vi "MT Detect FSK.vi"(5 "input complex waveform":T3={"t0"=0.0, "dt"=1.0, "Y"=[]} {"Y" format="%.3f"; "dt" format="%^.2e"; "t0" format="%.4f"}, 7 "FSK system parameters":T2={"samples per symbol (16)"=16, "symbol map"=[], "symbol phase continuity"=enum."continuous"} {"symbol map" format="%.2f"}, 9 "synchronization parameters":T1 {"sync sequence" format="%.2f"}, 11 "error in (no error)":errorcluster, 12 "matched filter coefficients":dbl[](array[numeric]) format="%.2f", 13 "reset? (T)":bool=TRUE, 14 "flush buffers? (F)":bool) -> (6 "output bit stream":i8[](array[numeric]), 10 "sync found index (symbols)":dbl format="%.4f", 15 "error out":errorcluster)   [LabVIEW 2020, in "niDMT.lvlib"]
doc: "Demodulates a frequency-shift keying (FSK)-modulated complex baseband waveform and returns the demodulated information bit stream. This VI attempts to remove carrier and phase offset by locking to the carrier signal."
uses:
  <vilib>/addons/Modulation/niDMT.lvlib
  <vilib>/addons/Modulation/Analog/controls/Complex Data Waveform.ctl
  <vilib>/Utility/error.llb/Error Cluster From Error Code.vi
  <vilib>/addons/Modulation/Digital/Support/Common/mod_Truncate FIR Filter (real).vi
  <vilib>/Analysis/NI_AALBase.lvlib
  <vilib>/addons/Modulation/niAMT.lvlib
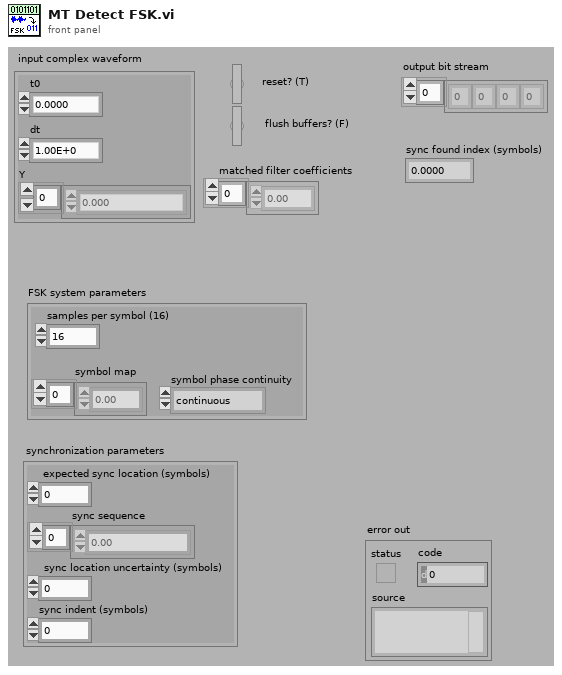
[diagram p1: front panel]
types:
  T1 = cluster{"expected sync location (symbols)":i32, "sync sequence":cdb[], "sync location uncertainty (symbols)":i32, "sync indent (symbols)":i32}
  T2 = cluster{"samples per symbol (16)":i32, "symbol map":dbl[], "symbol phase continuity":enum16{"continuous", "discontinuous"}}
  T3 = typedef "niAMT.lvlib/Complex Data Waveform.ctl" = cluster{"t0":dbl, "dt":dbl, "Y":cdb[]}
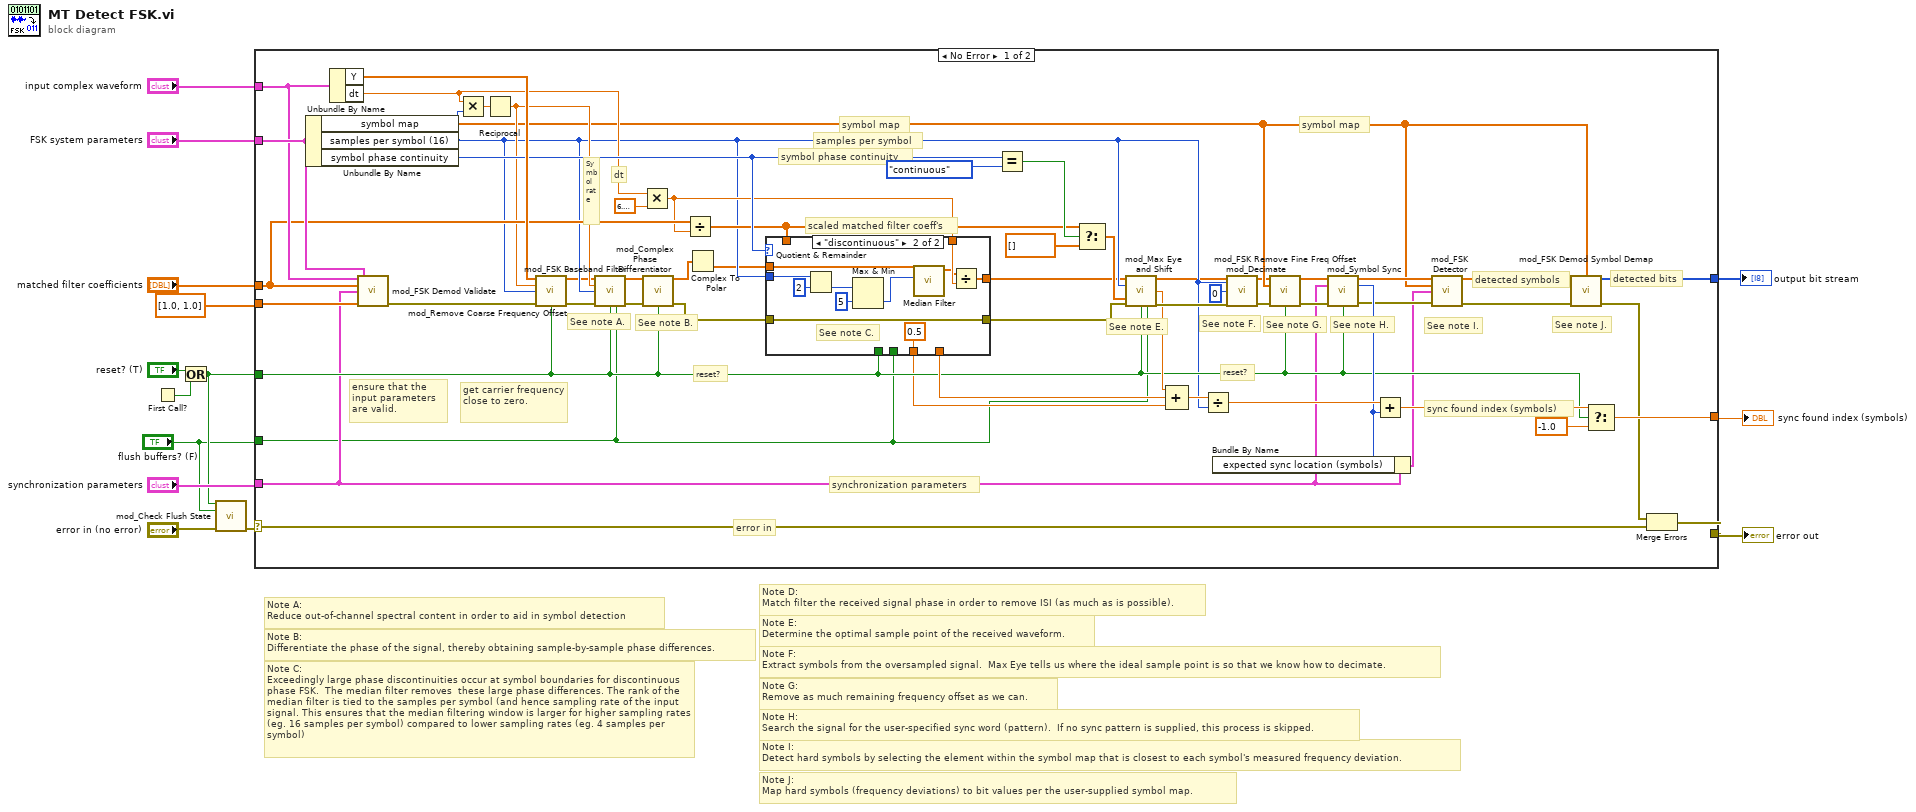
[diagram p0: block diagram]
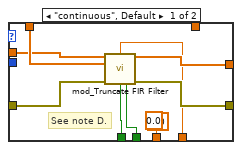
[diagram p2: hidden frame]
diagram:
  # "Note J:\nMap hard symbols (frequency deviations) to bit values per the user-supplied symbol map."
  # "Note I:\nDetect hard symbols by selecting the element within the symbol map that is closest to each symbol's measured frequency deviation."
  # "Note H:\nSearch the signal for the user-specified sync word (pattern).  If no sync pattern is supplied, this process is skipped."
  # "Note G:\nRemove as much remaining frequency offset as we can."
  # "Note F:\nExtract symbols from the oversampled signal.  Max Eye tells us where the ideal sample point is so that we know how to decimate."
  # "Note E:\nDetermine the optimal sample point of the received waveform."
  # "Note D:\nMatch filter the received signal phase in order to remove ISI (as much as is possible)."
  # "Note C:\nExceedingly large phase discontinuities occur at symbol boundaries for discontinuous phase FSK.  The median filter removes  these large phase differences. The rank of the \nmedian filter is tied to the samples per symbol (and hence sampling rate of the input\nsignal. This ensures that the median filtering window is larger for higher sampling rates\n(eg. 16 samples per symbol) compared to lower sampling rates (eg. 4 samples per symbol)"
  # "Note B:\nDifferentiate the phase of the signal, thereby obtaining sample-by-sample phase differences."
  # "Note A:\nReduce out-of-channel spectral content in order to aid in symbol detection"
  n1 = First Call?() -> (First Call?: T/F=w6:bool)
  n2 = Or(x="reset? (T)", y=w6) -> (x .or. y?=w3:bool)
  n3 = call <vilib>:"mod_Check Flush State.vi"("reset?"=w3, "flush buffers? (F)"="flush buffers? (F)", "error in (no error)"="error in (no error)") -> ("error out"=w4:errorcluster)  [unwired: 12 out]
  n4 = case shown="No Error" w4 {
    selector: w4 -> [w26 w91]
    tunnel: [w25 w91] -> w8
    tunnel: "synchronization parameters" -> [w24 _]
    tunnel: "matched filter coefficients" -> [w52 _]
    tunnel: "FSK system parameters" -> [w65 _]
    tunnel: dbl[] [1.0, 1.0] ("pulse shaping filter coefficients") -> [w57 _]
    tunnel: [w59 _] -> w9
    tunnel: "input complex waveform" -> [w54 _]
    tunnel: [w69 _] -> w10
    tunnel: w3 -> [w37 _]
    tunnel: "flush buffers? (F)" -> [w16 _]
    frame No Error {
      # "See note I."
      # "Symbol rate"
      # "See note J."
      # "See note H."
      # "See note G."
      # "See note F."
      # "See note E."
      # "get carrier frequency close to zero."
      # "ensure that the input parameters are valid."
      # "See note B."
      # "See note A."
      # "detected bits"
      # "error in"
      # "synchronization parameters"
      # "sync found index (symbols)"
      # "reset?"
      # "reset?"
      # "detected symbols"
      # "symbol map"
      # "dt"
      # "scaled matched filter coeff's"
      # "symbol phase continuity"
      # "samples per symbol"
      # "symbol map"
      # "dt"
      n5 = Unbundle By Name(w65) -> ("symbol map"=w34:dbl[], "samples per symbol (16)"=w29:i32, "symbol phase continuity"=w47:enum16{"continuous", "discontinuous"})
      n6 = Unbundle By Name(w54) -> ("Y"=w67:cdb[], "dt"=w39:dbl)
      n7 = call <vilib>:"mod_FSK Demod Validate.vi"("Input Complex Waveform"=w54, "FSK System Parameters"=w65, "Matched Filter Coefficients"=w52, "Synchronization Parameters"=w24, "Pulse Shaping Filter Coefficients"=w57) -> ("error out"=w66:errorcluster)  [unwired: 10 out]
      n8 = Multiply(x=w39, y=w29) -> (x*y=w68:dbl)
      n9 = Reciprocal(x=w68) -> (1/x=w38:dbl)
      n10 = call <vilib>:"mod_Remove Coarse Frequency Offset.vi"("Signal In"=w67, "Symbol Rate, Hz"=w38, "Samples Per Symbol (16)"=w29, "error in (no error)"=w66, "Reset? (T)"=w37) -> ("Signal Out"=w23:cdb[], "error out"=w48:errorcluster)  [unwired: 9 out]
      n11 = call <vilib>:"mod_FSK Baseband Filter.vi"("Signal In"=w23, "Symbol Rate, Hz"=w38, "Samples Per Symbol (16)"=w29, "error in (no error)"=w48, "Reset? (T)"=w37, "flush buffers? (F)"=w16) -> ("Signal Out"=w22:cdb[], "error out"=w49:errorcluster)  [unwired: 8 out]
      n12 = Multiply(x=w39, y=6.283185307179586) -> (x*y=w46:dbl)
      n13 = call <vilib>:"mod_Complex Phase Differentiator.vi"("Signal In"=w22, "error in (no error)"=w49, "Reset? (T)"=w37) -> ("Signal Out"=w21:cdb[], "error out"=w28:errorcluster)  [unwired: 11 out]
      n14 = Divide(x=w52, y=w46) -> (x/y=w44:dbl[])
      n15 = Complex To Polar(r * e^(i*theta)=w21) -> (theta=w15:dbl[])  [unwired: 1 out]
      n16 = case shown="\"discontinuous\"" w47 {
        tunnel: [w79 w88] -> w56
        tunnel: [w78 w89] -> w19
        tunnel: [w77 _] -> w53
        tunnel: w44 -> [w76 _]
        tunnel: w28 -> [w75 w88]
        tunnel: w37 -> [w74 _]
        tunnel: w46 -> [_ w90]
        tunnel: [0.0 0.5] -> w30
        tunnel: w15 -> [w72 w81]
        tunnel: w29 -> [_ w80]
        tunnel: w16 -> [w71 _]
        frame "continuous", Default {
          (unwired) 0.0
          # "See note D."
          n17 = call-poly <vilib>:"mod_Truncate FIR Filter.vi"("Signal In"=w72, "Filter Coefficients"=w76, "error in (no error)"=w75, "Reset? (T)"=w74, "flush buffers? (F)"=w71) -> ("Fractional Delay (samples)"=w77:dbl, "Signal Out"=w78:dbl[], "error out"=w79:errorcluster)  [unwired: 8 out]
        }
        frame "discontinuous" {
          # "See note C."
          n18 = Quotient & Remainder(x=w80, y=2) -> (floor(x/y)=w83:i32)  [unwired: 1 out]
          n19 = Max & Min(x=w83, y=5) -> (min(x,y)=w85:i32)  [unwired: 1 out]
          n20 = call <vilib>:"Median Filter.vi"("left rank"=w85, "X"=w81) -> ("Filtered X"=w86:dbl[])  [unwired: 1 in, 8 out]
          n21 = Divide(x=w86, y=w90) -> (x/y=w89:dbl[])
        }
      }
      n22 = Equal?(x=w47, y=enum16{"continuous", "discontinuous"}."continuous") -> (x = y?=w45:bool)
      n23 = Select(t=w44, s=w45, f=dbl[] []) -> (s? t:f=w42:dbl[])
      n24 = call <vilib>:"mod_Max Eye and Shift.vi"("Signal In"=w19, "Samples Per Symbol (16)"=w29, "matched filter coefficients"=w42, "error in (no error)"=w56, "Reset? (T)"=w37, "flush buffers? (F)"=w16) -> ("Signal Out"=w20:cdb[], "Optimal Offset (in Samples)"=w41:dbl, "error out"=w70:errorcluster)  [unwired: 1 in, 6 out]
      n25 = Compound Arithmetic op=ADD(w41, w53, w30) -> (w55:dbl)
      n26 = Divide(x=w55, y=w29) -> (x/y=w62:dbl)
      n27 = call <vilib>:"mod_Decimate.vi"("Signal In"=w20, "Samples Per Symbol (16)"=w29, "Offset"=0, "error in (no error)"=w70) -> ("Signal Out"=w18:cdb[], "error out"=w64:errorcluster)  [unwired: 1 in, 9 out]
      n28 = call <vilib>:"mod_FSK Remove Fine Freq Offset.vi"("Symbols"=w18, "Symbol Map"=w34, "error in (no error)"=w64, "Reset? (T)"=w37) -> ("Symbols"=w17:dbl[], "error out"=w63:errorcluster)  [unwired: 1 in, 9 out]
      n29 = call <vilib>:"mod_Symbol Sync.vi"("Signal In"=w17, "Synchronization Parameters"=w24, "error in (no error)"=w63, "Reset? (T)"=w37) -> ("Signal Out"=w35:cdb[], "Sync Location (symbols)"=w61:i32, "error out"=w36:errorcluster)  [unwired: 9 out]
      n30 = Bundle By Name(cluster=w24, "expected sync location (symbols)"=w61) -> (w33:T1)
      n31 = Add(x=w62, y=w61) -> (x+y=w58:dbl)
      n32 = call <vilib>:"mod_FSK Detector.vi"("Symbols"=w35, "Symbol Map"=w34, "Synchronization Parameters"=w33, "error in (no error)"=w36) -> ("Detected Symbols"=w32:dbl[], "error out"=w31:errorcluster)  [unwired: 1 in, 9 out]
      n33 = call <vilib>:"mod_FSK Demod Symbol Demap.vi"("Symbols In"=w32, "Symbol Map"=w34, "error in (no error)"=w31) -> ("Bits Out"=w69:i8[], "error out"=w27:errorcluster)  [unwired: 11 out]
      n34 = Select(t=w58, s=w37, f=-1.0) -> (s? t:f=w59:dbl)
      n35 = Merge Errors(w27, w26) -> (w25:errorcluster)
    }
    frame Error {
    }
  }
  "error out" <- w8
  "sync found index (symbols)" <- w9
  "output bit stream" <- w10
